vi "Init.vi"(8 "error in (no error)":errorcluster, 11 "Domain_Evolut":refnum<class "NI_Domain_Evolut.lvclass">) -> (0 "error out":errorcluster, 3 "initialized Domain_Evolut":refnum<class "NI_Domain_Evolut.lvclass">)   [LabVIEW 2020, in "NI_PDE.lvlib" / "NI_Domain_Evolut.lvclass"]
uses:
  <vilib>/gmath/pde.llb/DomainClass/Domain_Evolut/NI_Domain_Evolut.lvclass
  <vilib>/gmath/pde.llb/DomainClass/Class Type.ctl
  <vilib>/gmath/pde.llb/DomainClass/Domain_Evolut/NI_Domain_Evolut.lvclass/NI_Domain_Evolut.ctl
  <vilib>/gmath/pde.llb/DomainClass/NI_Domain.lvclass
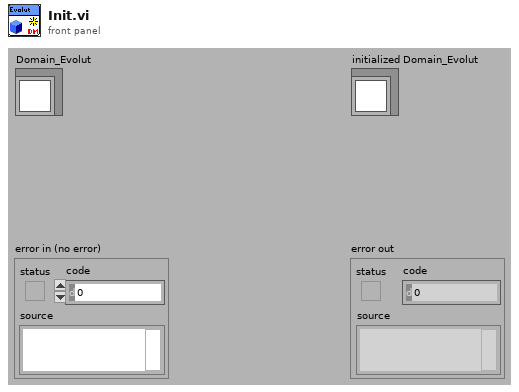
[diagram p1: front panel]
types:
  T1 = cluster{"start x":dbl, "end x":dbl, "# of x-points":i32}
  T2 = typedef "NI_PDE.lvlib/NI_Domain.lvclass/Class Type.ctl" = i32
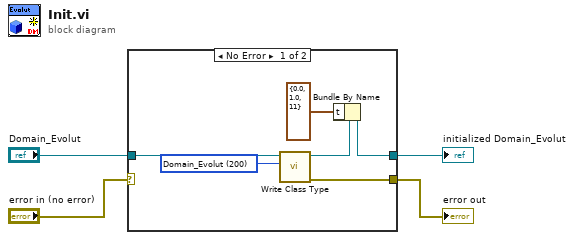
[diagram p0: block diagram]
diagram:
  n1 = case shown="No Error" "error in (no error)" {
    selector: "error in (no error)" -> [_ w12]
    tunnel: "Domain_Evolut" -> [w9 w11]
    tunnel: [w8 w12] -> w3
    tunnel: [w6 w11] -> w2
    frame No Error {
      w10 = T2 200 items=["Domain"=0, "Domain_Steady"=100, "Domain_Steady_2D_Rect"=121, "Domain_Steady_2D_Polygon"=122, "Domain_Evolut"=200, "Domain_Evolut_1D"=210, "Domain_Evolut_2D_Rect"=221] ("domain class type")
      n2 = call-dynamic "Write Class Type.vi"("domain class type"=w10, "Domain.lvclass in"=w9) -> ("error out"=w8:errorcluster, "Domain.lvclass out"=w7:refnum<class "NI_Domain_Evolut.lvclass">)  [unwired: 1 in, 7 out]
      n3 = Bundle By Name(cluster=w7, "t"=T1 {"start x"=0.0, "end x"=1.0, "# of x-points"=11} ("x")) -> (w6:refnum<class "NI_Domain_Evolut.lvclass">)
    }
    frame Error {
    }
  }
  "initialized Domain_Evolut" <- w2
  "error out" <- w3
